vi "tearDown.vi"(8 "error in (no error)":errorcluster, 11 "reference in":refnum<class "testcase-CSMSubModule.lvclass">) -> (0 "error out":errorcluster, 3 "reference out":refnum<class "testcase-CSMSubModule.lvclass">)   [LabVIEW 2017, in "testcase-CSMSubModule.lvclass"]
doc: "tearDown runs after the test method has completed. Use this method to clean up any operations or references that were opened by setUp or the test method. Unit tests should be independent of other unit tests so this VI should ensure that the next test can run in a 'clean' test environment."
uses:
  testcase-CSMSubModule.lvclass
  testcase-CSMSubModule.lvclass/testcase-CSMSubModule.ctl
  src/user.lib/_NEVSTOP/Communicable State Machine(CSM)/Communicable State Machine.lvlib
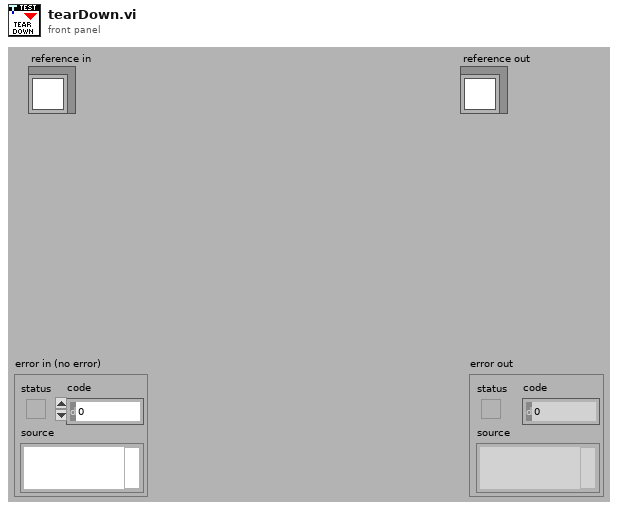
[diagram p1: front panel]
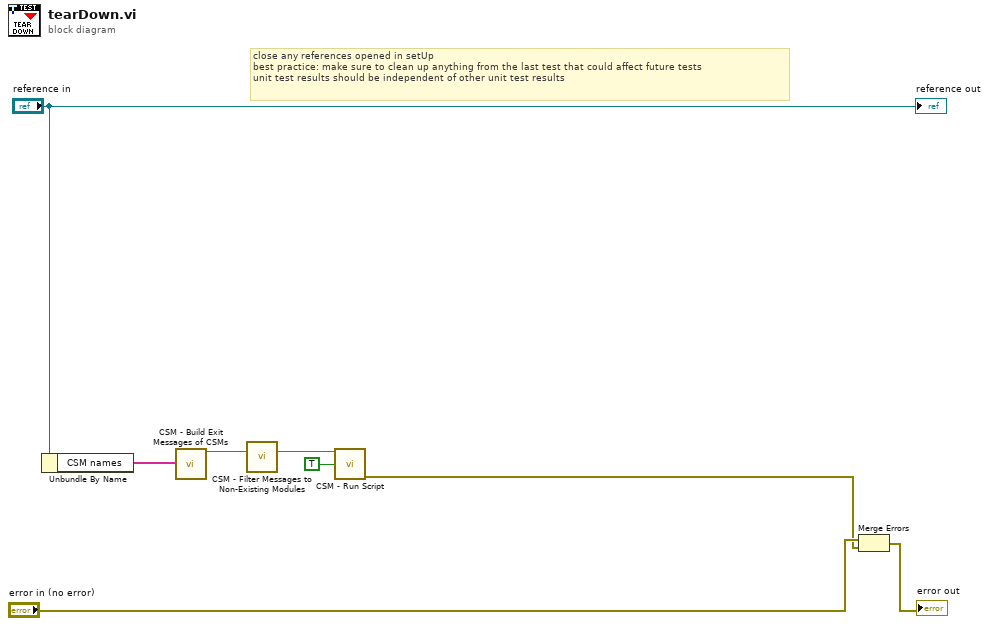
[diagram p0: block diagram]
diagram:
  # "close any references opened in setUp\nbest practice: make sure to clean up anything from the last test that could affect future tests\nunit test results should be independent of other unit test results"
  n1 = Unbundle By Name("reference in") -> ("CSM names"=w2:string[])
  n2 = call "CSM - Build Exit Messages of CSMs.vi"("CSMs"=w2) -> ("States"=w5:string)  [unwired: 14 in]
  n3 = call "CSM - Filter Messages to Non-Existing Modules.vi"("States In"=w5) -> ("States Out"=w3:string)  [unwired: 14 in]
  n4 = call "CSM - Run Script.vi"("CSM Scripts"=w3, "Continue If Error? (F)"=TRUE) -> ("error out"=w1:errorcluster)  [unwired: 11 in, 2 out]
  n5 = Merge Errors("error in (no error)", w1) -> (→"error out":errorcluster)
  "reference out" <- "reference in"
